vi "CHD_DRIVE_SET_GYRO.vi"(11 "Gyro Heading Radians":dbl) -> ()   [LabVIEW 2019]
uses:
  CHD_DRIVE_GLOBALS.vi
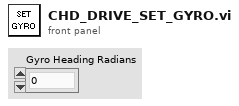
[diagram p1: front panel]
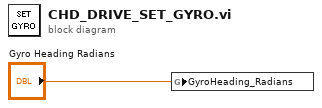
[diagram p0: block diagram]
diagram:
  n1 = global write "CHD_DRIVE_GLOBALS.vi" "GyroHeading_Radians"("Gyro Heading Radians") -> ()
